vi "ProcessTTRecHHT3.vi"(8 "oflcorr_in":u64, 11 "rawbits":u32) -> (0 "markercode":u32, 1 "is_marker":bool, 2 "channel":u32, 3 "dtime":u32, 4 "oflcorr_out":u64, 5 "numsync":u64, 7 "is_photon":bool)   [LabVIEW 2010]
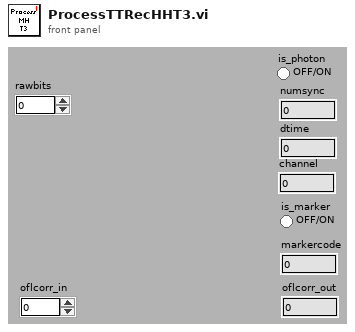
[diagram p1: front panel]
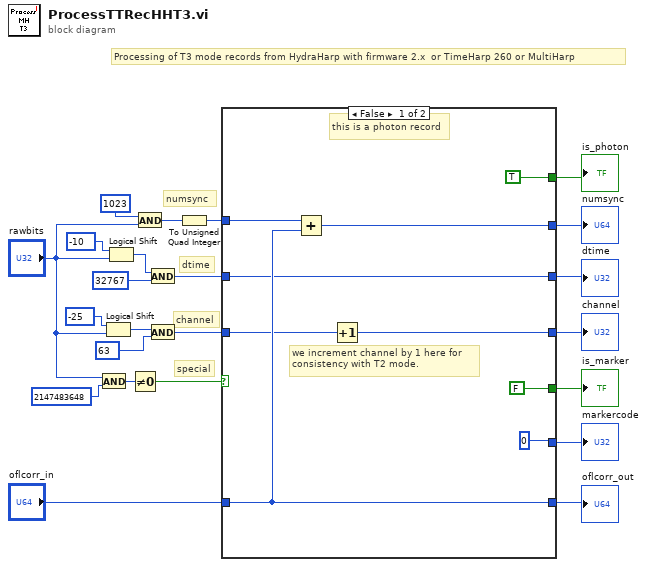
[diagram p0: block diagram]
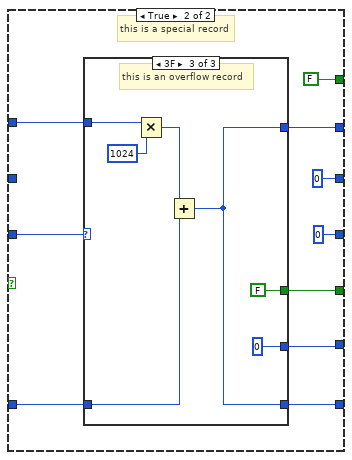
[diagram p2: hidden frame]
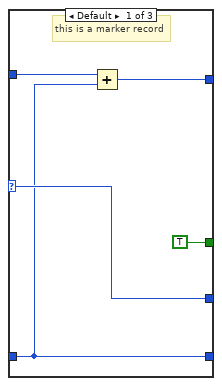
[diagram p3: hidden frame]
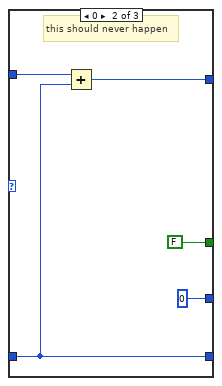
[diagram p4: hidden frame]
diagram:
  # "special"
  # "Processing of T3 mode records from HydraHarp with firmware 2.x  or TimeHarp 260 or MultiHarp"
  # "dtime"
  # "channel"
  # "numsync"
  n1 = And(x="rawbits", y=u32 2147483648 ("x")) -> (x .and. y?=w7:u32)
  n2 = Logical Shift(y=-25, x="rawbits") -> (x << y=w17:u32)
  n3 = Logical Shift(y=-10, x="rawbits") -> (x << y=w20:u32)
  n4 = Not Equal To 0?(x=w7) -> (x != 0?=w4:bool)
  n5 = And(x=u32 1023, y="rawbits") -> (x .and. y?=w2:u32)
  n6 = And(x=w20, y=u32 32767 ("x")) -> (x .and. y?=w18:u32)
  n7 = And(x=w17, y=u32 63 ("x")) -> (x .and. y?=w3:u32)
  n8 = To Unsigned Quad Integer(1:w2) -> (0:w1:u64)
  n9 = case shown="False" w4 {
    tunnel: w1 -> [w26 w33]
    tunnel: "oflcorr_in" -> [w29 w40]
    tunnel: [w29 w39] -> w14
    tunnel: [FALSE w37] -> w12
    tunnel: [u32 0 w38] -> w13
    tunnel: [TRUE FALSE] -> w10
    tunnel: w18 -> [w27 _]
    tunnel: [w28 w34] -> w9
    tunnel: [w27 u32 0] -> w8
    tunnel: [w24 u32 0] -> w11
    tunnel: w3 -> [w25 w36]
    frame False {
      # "we increment channel by 1 here for\nconsistency with T2 mode."
      # "this is a photon record"
      n10 = Add(x=w26, y=w29) -> (x+y=w28:u64)
      n11 = Increment(x=w25) -> (x+1=w24:u32)
    }
    frame True {
      # "this is a special record"
      n12 = case shown="3F" w36 {
        selector: w36 -> [w46 _ _]
        tunnel: w40 -> [w44 w49 w54]
        tunnel: [w44 w49 w53] -> w39
        tunnel: [TRUE FALSE FALSE] -> w37
        tunnel: [w46 u32 0 u32 0] -> w38
        tunnel: [w43 w48 w53] -> w34
        tunnel: w33 -> [w45 w50 w57]
        frame Default {
          # "this is a marker record"
          n13 = Add(x=w45, y=w44) -> (x+y=w43:u64)
        }
        frame 0 {
          # "this should never happen"
          n14 = Add(x=w50, y=w49) -> (x+y=w48:u64)
        }
        frame 63 {
          # "this is an overflow record"
          n15 = Multiply(x=w57, y=u64 1024 ("x")) -> (x*y=w55:u64)
          n16 = Add(x=w55, y=w54) -> (x+y=w53:u64)
        }
      }
    }
  }
  "channel" <- w11
  "numsync" <- w9
  "is_photon" <- w10
  "markercode" <- w13
  "is_marker" <- w12
  "oflcorr_out" <- w14
  "dtime" <- w8
